vi "StateMachine1.vi"() -> ()   [LabVIEW 2018]
panel:
  in  "Dur_ms":u32
  in  "Toggle":bool
  out "Waveform Chart":dbl(graph)
  out "Boolean":bool
  out "Text Data":string
  in  "String":string
  in  "Clear":bool
  in  "Set":bool
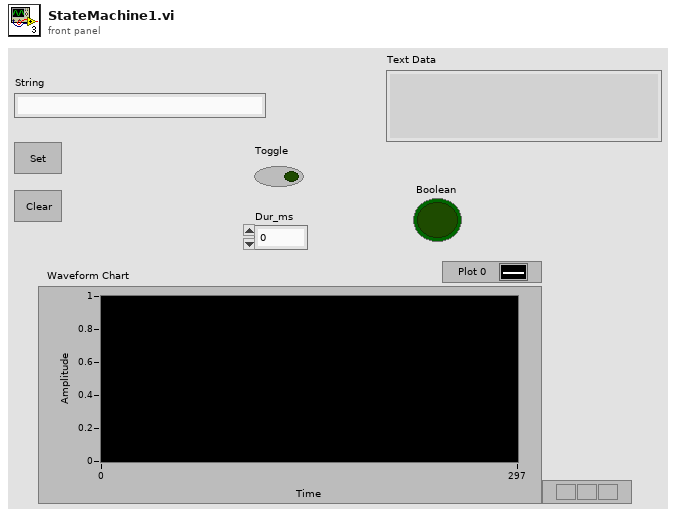
[diagram p1: front panel]
types:
  T1 = cluster{"Duration":u32, "State":bool, "Running":bool}
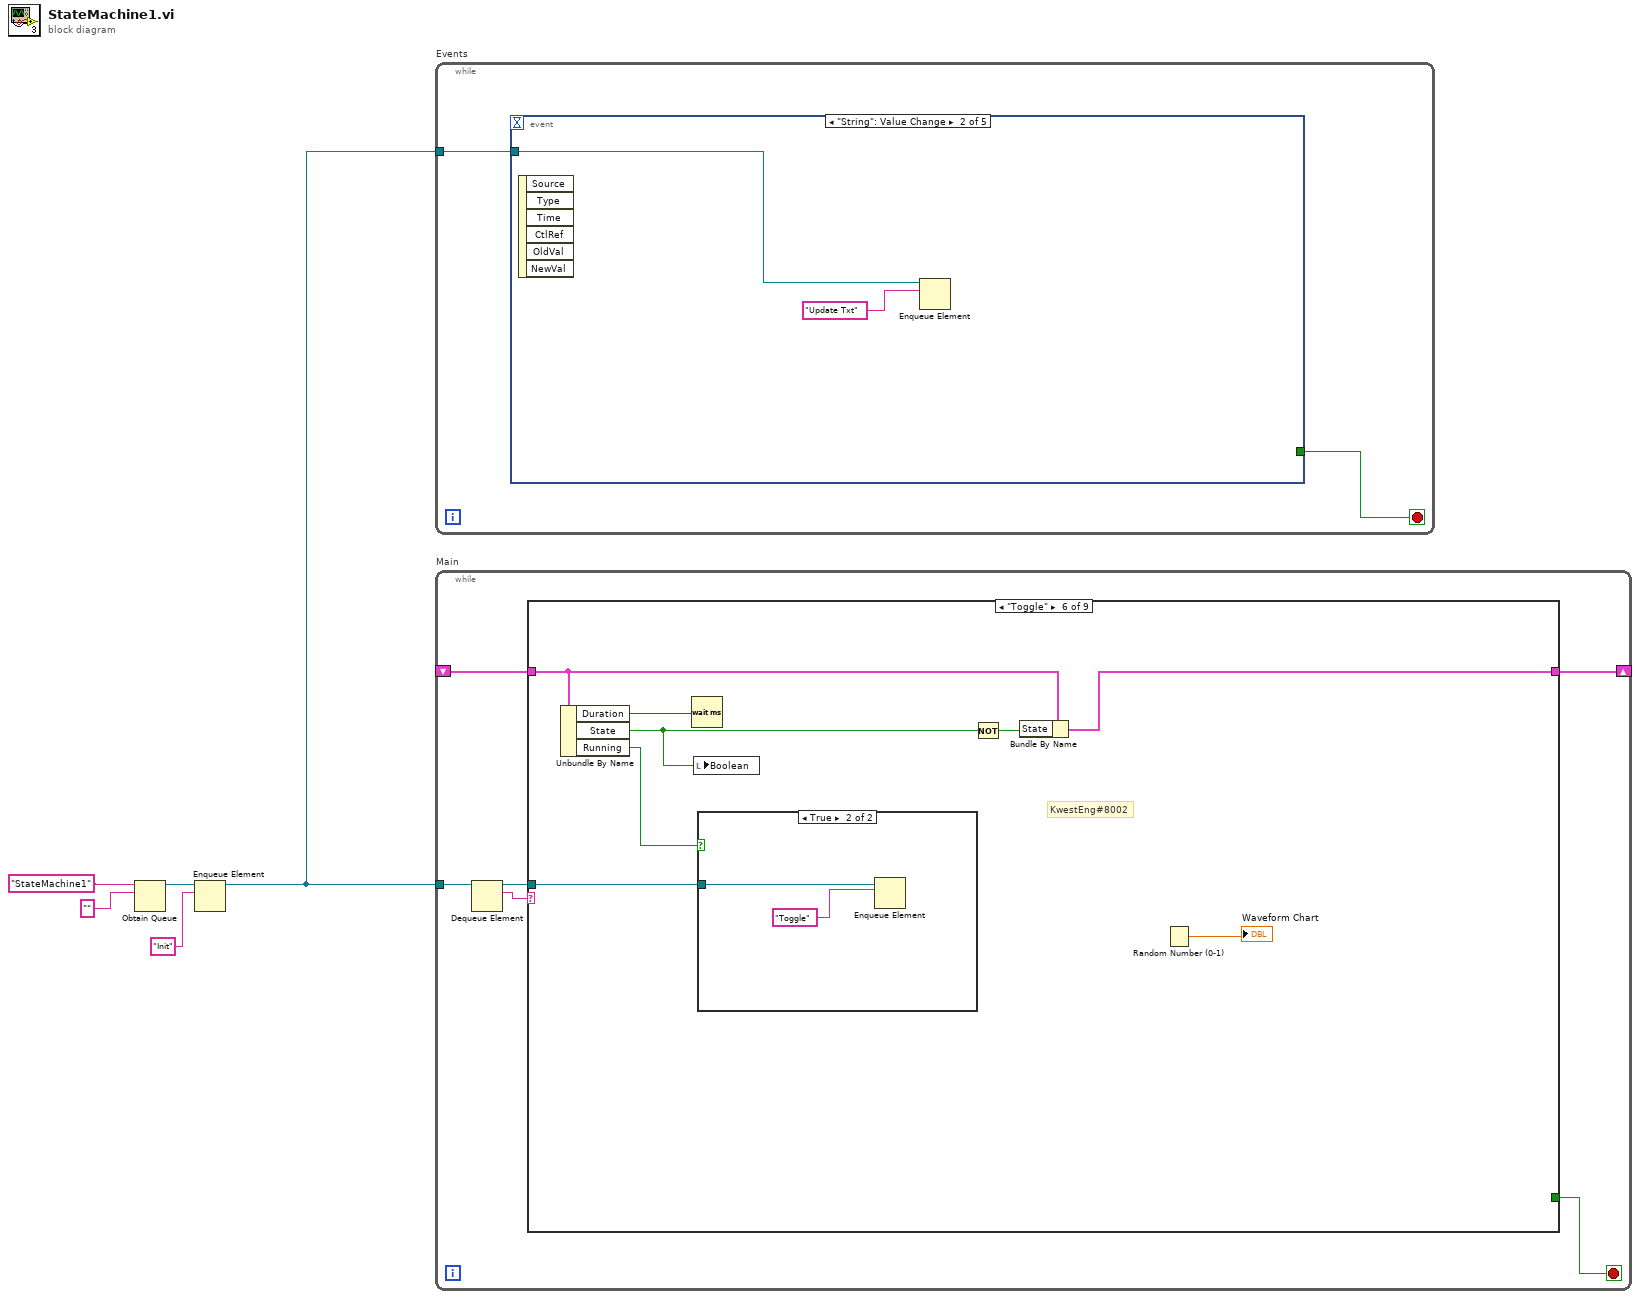
[diagram p0: block diagram]
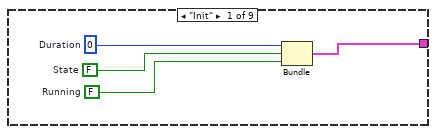
[diagram p2: hidden frame]
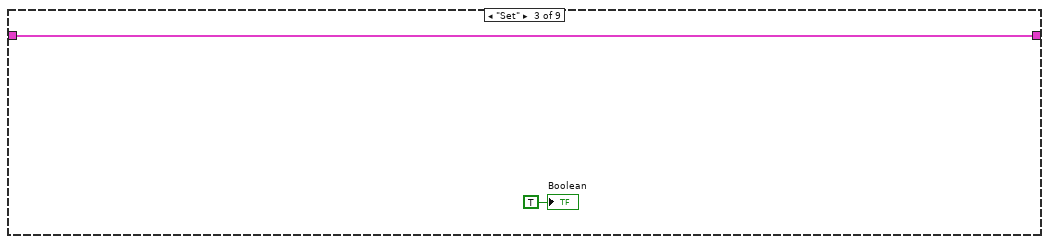
[diagram p4: hidden frame]
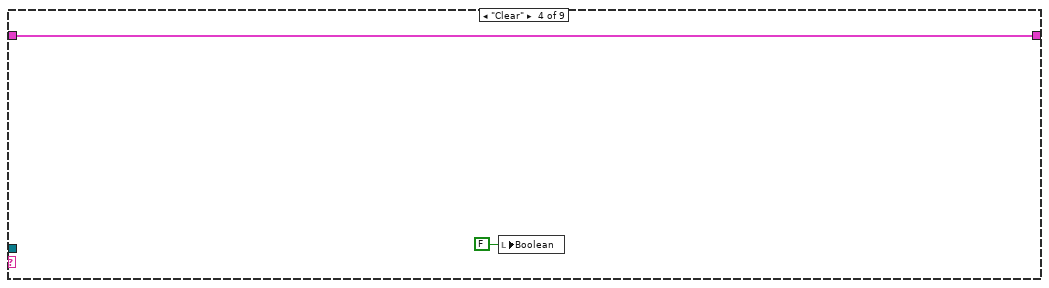
[diagram p5: hidden frame]
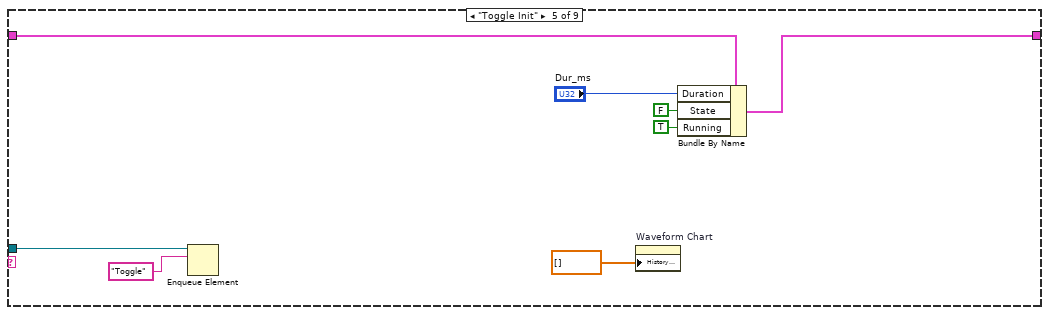
[diagram p6: hidden frame]
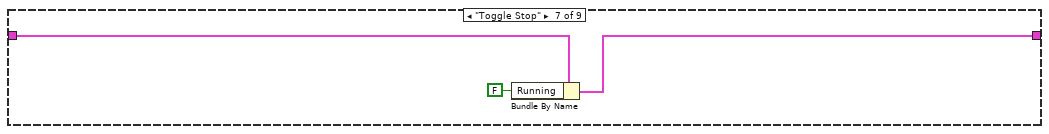
[diagram p8: hidden frame]
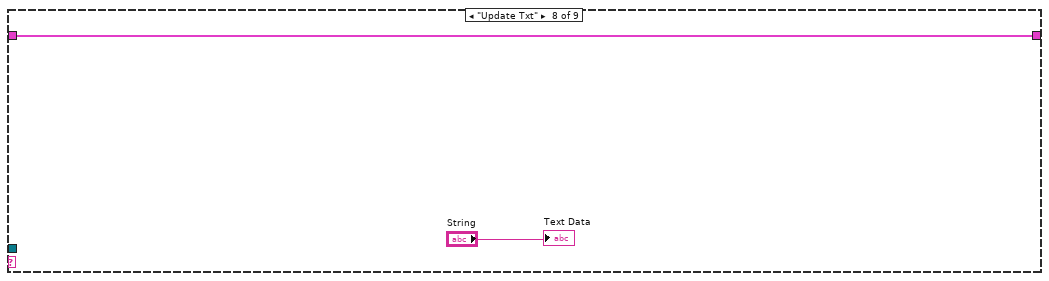
[diagram p9: hidden frame]
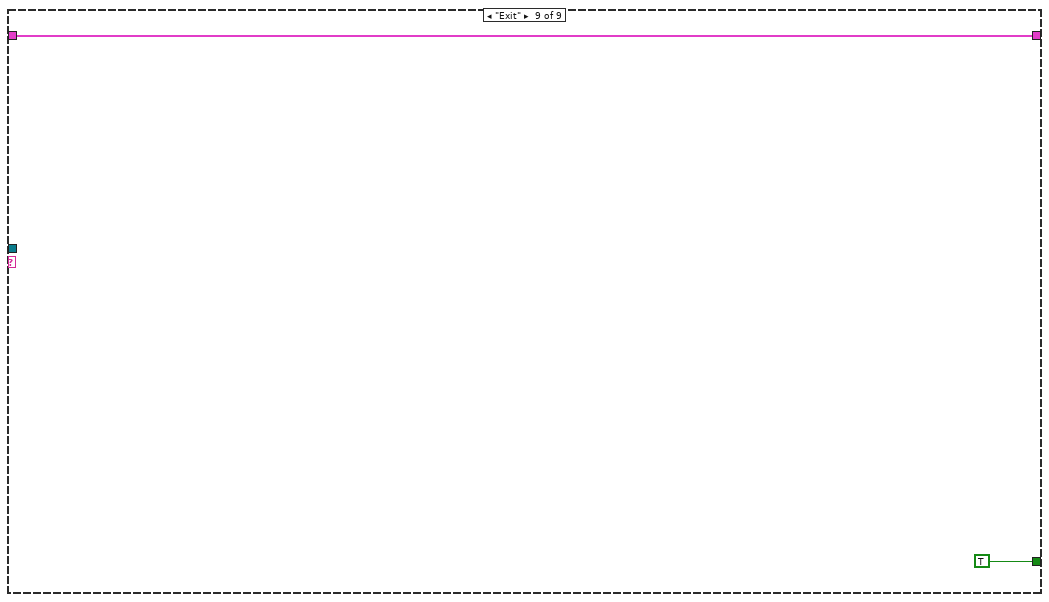
[diagram p10: hidden frame]
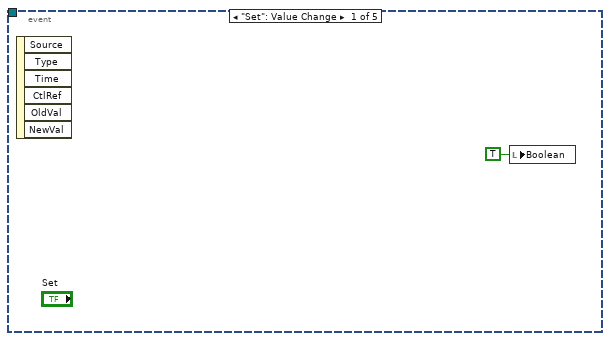
[diagram p11: hidden frame]
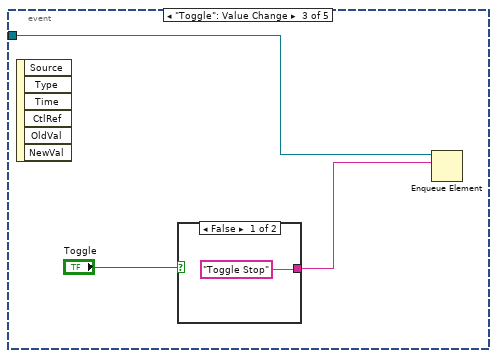
[diagram p12: hidden frame]
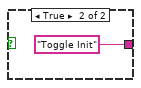
[diagram p13: hidden frame]
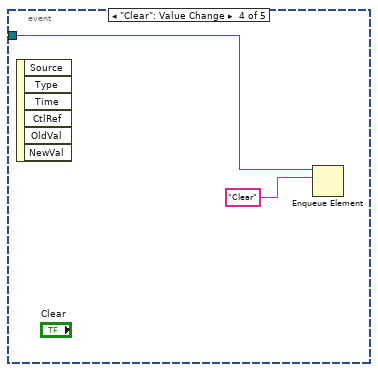
[diagram p14: hidden frame]
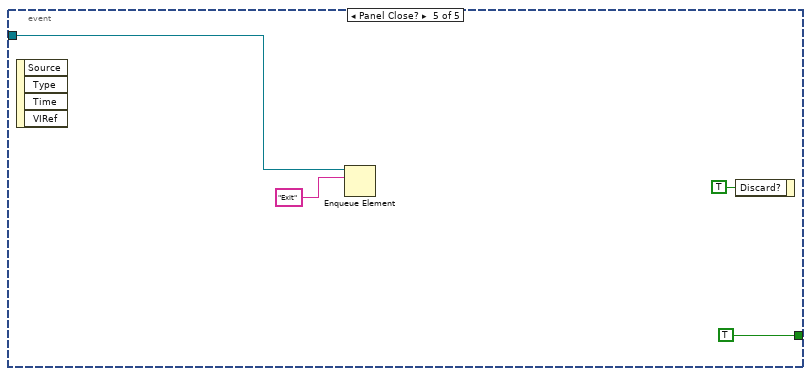
[diagram p15: hidden frame]
diagram:
  n1 = Obtain Queue(name (unnamed)="StateMachine1", element data type="") -> (queue out=w3:refnum<queue>)  [unwired: 3 in, 2 out]
  n2 = Enqueue Element(queue=w3, element="Init") -> (queue out=w2:refnum<queue>)  [unwired: 2 in, 2 out]
  n3 = while "Events" {
    tunnel: w2 -> [w7]
    stop <- w6 stop-if-true
    n4 = event shown="[1] \"String\": Value Change" {
      selector: _ -> [_ _ _ _ _]
      dyn-events: _ -> [_ _ _ _ _]
      timeout: _ -> [_ _ _ _ _]
      tunnel: w7 -> [_ w9 w13 w17 w19]
      tunnel: [_ _ _ _ TRUE] -> w6
      event "Set": Value Change {
        n5 = event-data() -> ()  [unwired: 1 in, 6 out]
        n6 = local write "Boolean"(TRUE ("Boolean")) -> ()
      }
      event "String": Value Change {
        n7 = event-data() -> ()  [unwired: 1 in, 6 out]
        n8 = Enqueue Element(queue=w9, element="Update Txt") -> ()  [unwired: 2 in, 3 out]
      }
      event "Toggle": Value Change {
        n9 = event-data() -> ()  [unwired: 1 in, 6 out]
        n10 = case shown="False" "Toggle" {
          tunnel: ["Toggle Stop" ("element") "Toggle Init" ("element")] -> w11
          frame False {
          }
          frame True {
          }
        }
        n11 = Enqueue Element(queue=w13, element=w11) -> ()  [unwired: 2 in, 3 out]
      }
      event "Clear": Value Change {
        n12 = event-data() -> ()  [unwired: 1 in, 6 out]
        n13 = Enqueue Element(queue=w17, element="Clear") -> ()  [unwired: 2 in, 3 out]
      }
      event Panel Close? {
        n14 = event-data() -> ()  [unwired: 1 in, 4 out]
        n15 = Enqueue Element(queue=w19, element="Exit") -> ()  [unwired: 2 in, 3 out]
        n16 = event-data("Discard?"=TRUE) -> ()  [unwired: 1 in, 1 out]
      }
    }
  }
  n17 = while "Main" {
    tunnel: w2 -> [w27]
    shift-right: [w22] -> _
    shift-left: _ -> [w23]
    stop <- w24 stop-if-true
    n18 = Dequeue Element(queue=w27) -> (queue out=w25:refnum<queue>, element=w26:string)  [unwired: 2 in, 2 out]
    n19 = case shown="\"Toggle\"" w26 {
      tunnel: w25 -> [_ _ _ _ w40 w52 _ _ _]
      tunnel: [_ _ _ _ _ _ _ _ TRUE] -> w24
      tunnel: w23 -> [_ w32 w33 w35 w41 w50 w55 w59 w60]
      tunnel: [w31 w32 w33 w35 w42 w47 w56 w59 w60] -> w22
      frame "Init" {
        w28 = FALSE  # Running
        w29 = FALSE  # State
        w30 = u32 0  # Duration
        n20 = Bundle("Duration"=w30, "State"=w29, "Running"=w28) -> (w31:T1)  [unwired: 1 in]
      }
      frame Default {
      }
      frame "Set" {
        "Boolean" <- TRUE ("Boolean")
      }
      frame "Clear" {
        n21 = local write "Boolean"(FALSE ("Boolean")) -> ()
      }
      frame "Toggle Init" {
        n22 = Enqueue Element(queue=w40, element="Toggle") -> ()  [unwired: 2 in, 3 out]
        n23 = property on="Waveform Chart" class="WFChart (strict)"("History Data"=dbl[] []) -> ()  [unwired: 2 in, 2 out]
        n24 = Bundle By Name(cluster=w41, "Duration"="Dur_ms", "State"=FALSE, "Running"=TRUE) -> (w42:T1)
      }
      frame "Toggle" {
        # "KwestEng#8002"
        n25 = Unbundle By Name(w50) -> ("Duration"=w51:u32, "State"=w48:bool, "Running"=w46:bool)
        n26 = Wait (ms)(milliseconds to wait=w51) -> ()  [unwired: 1 out]
        n27 = local write "Boolean"(w48) -> ()
        n28 = case shown="True" w46 {
          tunnel: w52 -> [_ w53]
          frame False {
          }
          frame True {
            n29 = Enqueue Element(queue=w53, element="Toggle") -> ()  [unwired: 2 in, 3 out]
          }
        }
        n30 = Not(x=w48) -> (.not. x?=w49:bool)
        n31 = Bundle By Name(cluster=w50, "State"=w49) -> (w47:T1)
        n32 = Random Number (0-1)() -> (number: 0 to 1=→"Waveform Chart":dbl)
      }
      frame "Toggle Stop" {
        n33 = Bundle By Name(cluster=w55, "Running"=FALSE) -> (w56:T1)
      }
      frame "Update Txt" {
        "Text Data" <- "String"
      }
      frame "Exit" {
      }
    }
  }
